vi "AMI_Compara_Max_Indices.vi"() -> (1 "Max_idx":i16, 6 "idxScanVf":i16, 8 "idxScanTf":i16, 9 "idxScanXf":i16, 10 "idxScanYf":i16, 11 "idxScanZf":i16)   [LabVIEW 2017]
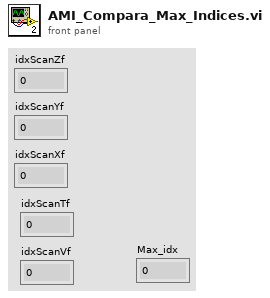
[diagram p1: front panel]
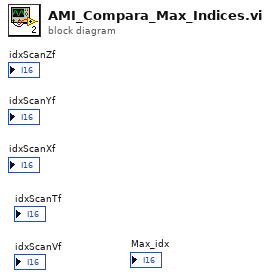
[diagram p0: block diagram]
diagram:
